vi "Configurable PWM Tester.vi"() -> ()   [LabVIEW 2021]
uses:
  <vilib>/Utility/error.llb/DialogType.ctl
  <vilib>/DAQmx/write.llb/DAQmx Write (Counter Frequency 1Chan 1Samp).vi
  <vilib>/DAQmx/create/channels.llb/DAQmx Create Channel (CO-Pulse Generation-Frequency).vi
  <vilib>/DAQmx/configure/timing.llb/DAQmx Timing (Implicit).vi
  <vilib>/DAQmx/miscellaneous.llb/DAQmx Fill In Error Info.vi
  <resource>/objmgr/daqmx.rc
panel:
  in  "duty cycle":dbl=0.1 min=0.05 max=0.1 format="%_6g"
  in  "stop":bool
  in  "Output Terminal":tag="/Dev1/PFI12"
  in  "Counter":tag="Dev1/ctr0"
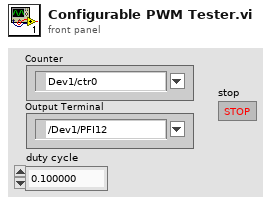
[diagram p1: front panel]
types:
  T1 = typedef "DialogType.ctl" = u16
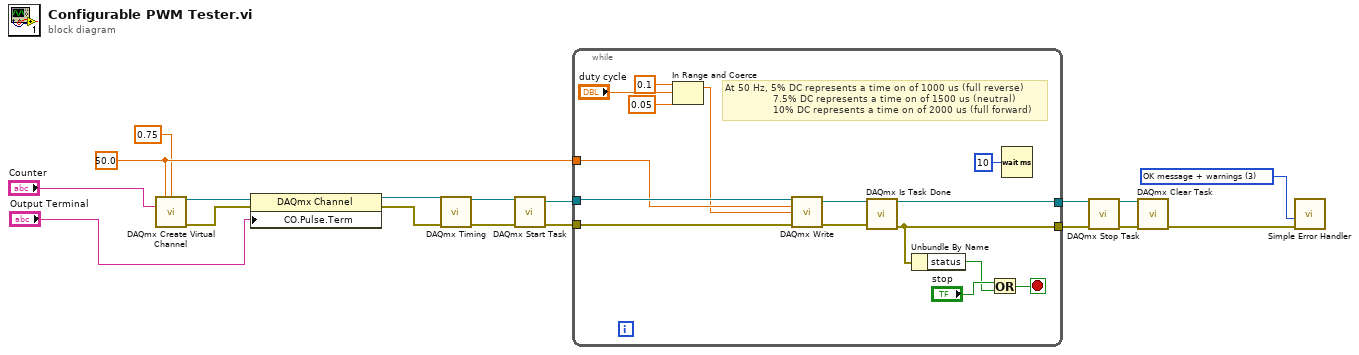
[diagram p0: block diagram]
diagram:
  w7 = 50.0 ("Frequency")
  w15 = T1 3 items=["no dialog", "OK message", "continue or stop message", "OK message + warnings", "continue/stop + warnings"] ("type of dialog (OK msg:1)")
  n1 = call-poly <vilib>:"DAQmx Create Virtual Channel.vi"("frequency"=w7, "duty cycle"=0.75, "counter"="Counter") -> ("task out"=w5:refnum<k21>, "error out"=w4:errorcluster)  [unwired: 11 in]
  n2 = property class="DAQmx Channel"(reference=w5, error in=w4, "CO.Pulse.Term"="Output Terminal") -> (reference out=w3:refnum<k21>, error out=w2:errorcluster)
  n3 = call-poly <vilib>:"DAQmx Timing.vi"("task/channels in"=w3, "error in"=w2) -> ("task out"=w10:refnum<k21>, "error out"=w9:errorcluster)  [unwired: 12 in]
  n4 = call <vilib>:"DAQmx Start Task.vi"("task/channels in"=w10, "error in"=w9) -> ("task out"=w13:refnum<k21>, "error out"=w12:errorcluster)  [unwired: 12 in]
  n5 = while {
    tunnel: w12 -> [w27]
    tunnel: [w30] -> w14
    tunnel: w13 -> [w26]
    tunnel: [w29] -> w11
    tunnel: w7 -> [w25]
    stop <- w32 stop-if-true
    # "At 50 Hz, 5% DC represents a time on of 1000 us (full reverse)\n                7.5% DC represents a time on of 1500 us (neutral)\n                10% DC represents a time on of 2000 us (full forward)"
    n6 = In Range and Coerce(upper limit=0.1, x="duty cycle", lower limit=0.05) -> (coerced(x)=w19:dbl)  [unwired: 1 out]
    n7 = call-poly <vilib>:"DAQmx Write.vi"("task/channels in"=w26, "frequency"=w25, "duty cycle"=w19, "error in"=w27) -> ("task out"=w23:refnum<k21>, "error out"=w24:errorcluster)  [unwired: 9 in, 1 out]
    n8 = call <vilib>:"DAQmx Is Task Done.vi"("task/channels in"=w23, "error in"=w24) -> ("task out"=w30:refnum<k21>, "error out"=w29:errorcluster)  [unwired: 11 in, 1 out]
    n9 = Unbundle By Name(w29) -> ("status"=w31:bool)
    n10 = Or(x="stop", y=w31) -> (x .or. y?=w32:bool)
    n11 = Wait (ms)(milliseconds to wait=u32 10) -> ()  [unwired: 1 out]
  }
  n12 = call <vilib>:"DAQmx Stop Task.vi"("task/channels in"=w14, "error in"=w11) -> ("task out"=w17:refnum<k21>, "error out"=w16:errorcluster)  [unwired: 12 in]
  n13 = call <vilib>:"DAQmx Clear Task.vi"("task in"=w17, "error in"=w16) -> ("error out"=w18:errorcluster)  [unwired: 13 in]
  n14 = call <vilib>:"Simple Error Handler.vi"("type of dialog (OK msg:1)"=w15, "error in (no error)"=w18) -> ()  [unwired: 3 in, 5 out]
